vi "Register Groups.vi"(8 "error in (no error)":errorcluster, 11 "DataLoggerAPI in":refnum<class "DataLoggerAPI.lvclass">) -> (0 "error out":errorcluster, 3 "DataLoggerAPI out":refnum<class "DataLoggerAPI.lvclass">)   [LabVIEW 2020, in "VolatusDataLogger.lvlib" / "DataLoggerAPI.lvclass"]
uses:
  DataLoggerAPI.lvclass
  DataLoggerAPI.lvclass/DataLoggerAPI.ctl
  DataLogger Messages/Register Groups Msg/Register Groups Msg.lvclass
  lv-promises/Promises/Promise/Promise.lvclass
  lv-promises/Promises/Error Result/Error Result.lvclass
  C:/dev/lv20CE/relink/lv-promises/Promises/Value/Value.lvclass
  C:/dev/lv20CE/relink/lv-promises/Promises/Error Result/Error Result.lvclass
  lv-promises/Promises/Future/Future.lvclass
  lv-vecto/Vecto/Group/Group.lvclass
panel:
  in  "Groups":refnum<class "Group.lvclass">[](array[class])
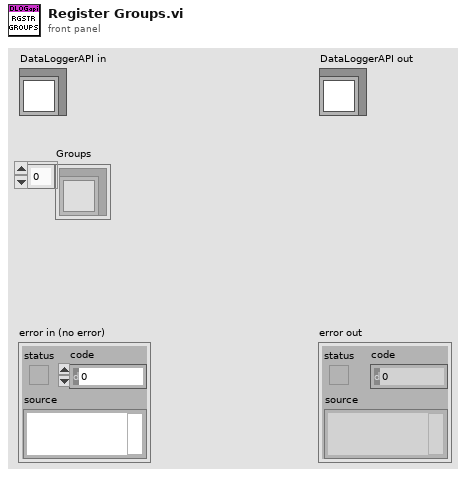
[diagram p1: front panel]
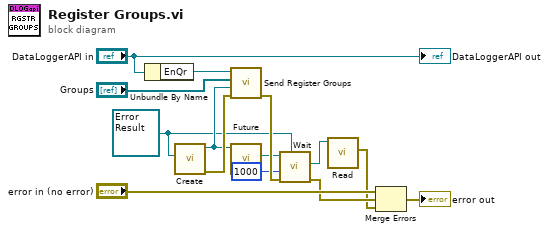
[diagram p0: block diagram]
diagram:
  w7 = refnum<class "Error Result.lvclass"> refnum ("Futures:Error Result.lvclass")
  n1 = Unbundle By Name("DataLoggerAPI in") -> ("EnQr"=w11:refnum<class "Message Enqueuer.lvclass">)
  n2 = call "Create.vi"("Result Type"=w7) -> ("error out"=w10:errorcluster, "Promise"=w9:refnum<class "Promise.lvclass">)  [unwired: 9 in]
  n3 = call "Send Register Groups.vi"("error in (no error)"=w10, "Promise"=w9, "Groups"="Groups", "Message Enqueuer"=w11) -> ("error out"=w14:errorcluster)  [unwired: 6 in, 1 out]
  n4 = call "Future.vi"("Promise in"=w9) -> ("Future"=w8:refnum<class "Future.lvclass">)  [unwired: 9 in, 1 out]
  n5 = call "Wait.vi"("Result Type"=w7, "error in (no error)"=w14, "Timeout mS (-1)"=1000, "Future in"=w8) -> ("error out"=w3:errorcluster, "Result"=w5:refnum<class "Error Result.lvclass">)  [unwired: 6 in]
  n6 = call "Read.vi"("Error Result in"=w5) -> ("Error"=w2:errorcluster)  [unwired: 10 in]
  n7 = Merge Errors("error in (no error)", w3, w2) -> (→"error out":errorcluster)
  "DataLoggerAPI out" <- "DataLoggerAPI in"
